vi "latch.vi"() -> ()   [LabVIEW 2011]
panel:
  in  "VariableToChange":bool
  out "Joyout":bool
  in  "JoyValue":bool
  out "ms":dbl
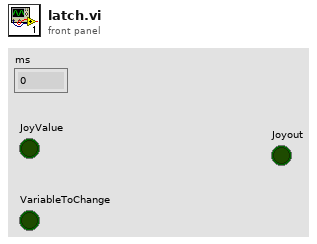
[diagram p1: front panel]
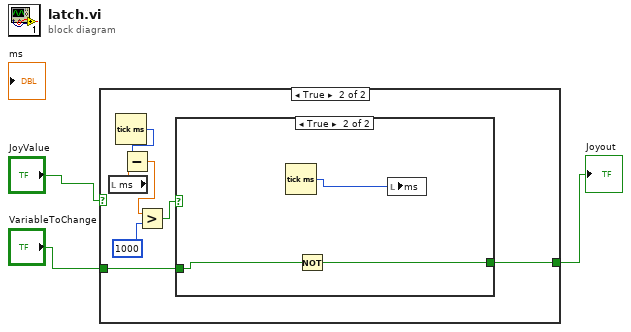
[diagram p0: block diagram]
diagram:
  n1 = case shown="True" "JoyValue" {
    tunnel: "VariableToChange" -> [w4 w6]
    tunnel: [w4 w5] -> w1
    frame False {
    }
    frame True {
      n2 = local read "ms"() -> (w10:dbl)
      n3 = Tick Count (ms)() -> (millisecond timer value=w11:u32)
      n4 = Subtract(x=w11, y=w10) -> (x-y=w9:dbl)
      n5 = Greater?(x=w9, y=1000) -> (0:w7:bool)
      n6 = case shown="True" w7 {
        tunnel: w6 -> [w12 w15]
        tunnel: [w12 w14] -> w5
        frame False {
        }
        frame True {
          n7 = Tick Count (ms)() -> (millisecond timer value=w13:u32)
          n8 = Not(x=w15) -> (.not. x?=w14:bool)
          n9 = local write "ms"(w13) -> ()
        }
      }
    }
  }
  "Joyout" <- w1
